vi "RampGenerator.vi"(2 "Number of Positions":u16=100 min=1 step=1, 3 "End  (um)":dbl=10.0 min=0.0 max=100.0 step=0.2 format="%.3f", 4 "Start  (um)":dbl=150.0 min=0.0 max=300.0 step=0.5 format="%.3f") -> (0 "Array":dbl[](array[numeric]) format="%.2f")   [LabVIEW 2019]
panel:
  # "Generates a linear ramp from Start to End (inclusive).\nThis example is used as a SubVI in the provided scanning examples."
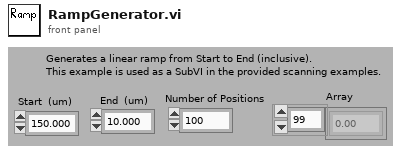
[diagram p1: front panel]
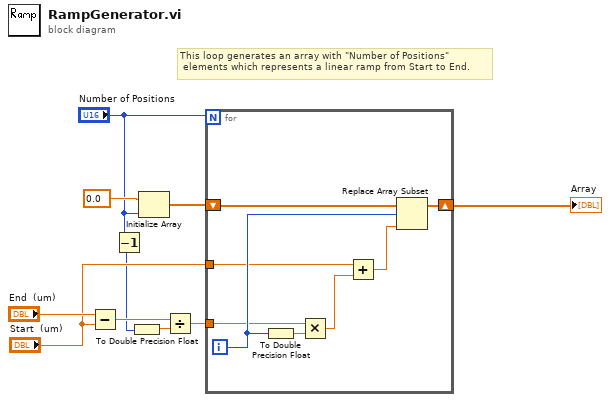
[diagram p0: block diagram]
diagram:
  # "This loop generates an array with \"Number of Positions\"\n elements which represents a linear ramp from Start to End."
  n1 = Subtract(x="End  (um)", y="Start  (um)") -> (x-y=w7:dbl)
  n2 = Decrement(x="Number of Positions") -> (x-1=w1:u16)
  n3 = To Double Precision Float(number=w1) -> (double precision float=w6:dbl)
  n4 = Initialize Array(0.0, "Number of Positions") -> (w9:dbl[])
  n5 = Divide(x=w7, y=w6) -> (x/y=w5:dbl)
  n6 = for {
    N: "Number of Positions" -> [_]
    shift-right: [w17] -> w4
    shift-left: w9 -> [w18]
    tunnel: w5 -> [w14]
    tunnel: "Start  (um)" -> [w11]
    i -> [w15]
    n7 = To Double Precision Float(number=w15) -> (double precision float=w16:dbl)
    n8 = Multiply(x=w14, y=w16) -> (x*y=w13:dbl)
    n9 = Add(x=w11, y=w13) -> (x+y=w12:dbl)
    n10 = Replace Array Subset(array=w18, new element=w12, index=w15) -> (w17:dbl[])
  }
  "Array" <- w4
